vi "SetHeight.vi"(10 "Height":dbl, 11 "Square In":refnum<class "Square.lvclass">) -> (3 "Square Out":refnum<class "Square.lvclass">)   [LabVIEW 2018, in "Square.lvclass"]
uses:
  Square.lvclass
  Rectangle/Rectangle.lvclass
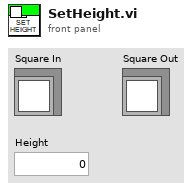
[diagram p1: front panel]
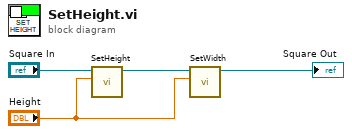
[diagram p0: block diagram]
diagram:
  n1 = call-parent "SetHeight.vi"("Height"="Height", "Rectangle In"="Square In") -> ("Rectangle Out"=w3:refnum<class "Square.lvclass">)  [unwired: 9 in]
  n2 = call-dynamic "SetWidth.vi"("Width"="Height", "Rectangle In"=w3) -> ("Rectangle Out"=→"Square Out":refnum<class "Square.lvclass">)  [unwired: 9 in]
